vi "Pass Ref and Receive Data.vi"(7 "Enum State":T1=enum."Pass Data", 8 "error in (no error)":errorcluster, 10 "Data":T2={"Raw Data"=[], "Volt Channel"={"Index"=[], "Chl Name"=[], "Scale"=[], "Offset"=[], "Sample Rate"=100, "Device Name"="", "Channel"=""}}, 11 "Graph Manager in":refnum<class "Display Abstract.lvclass">) -> (0 "error out":errorcluster, 2 "Data Out":waveform(dbl)[](array[waveform]), 3 "Graph Manager out":refnum<class "Display Abstract.lvclass">)   [LabVIEW 2021, in "Display Abstract.lvclass"]
doc: "Do nothing."
uses:
  Display Abstract.lvclass
  Graph Data -- cluster.ctl
  Control/Volt Chl.ctl
  Pass Ref and Receive Data -- Enum.ctl
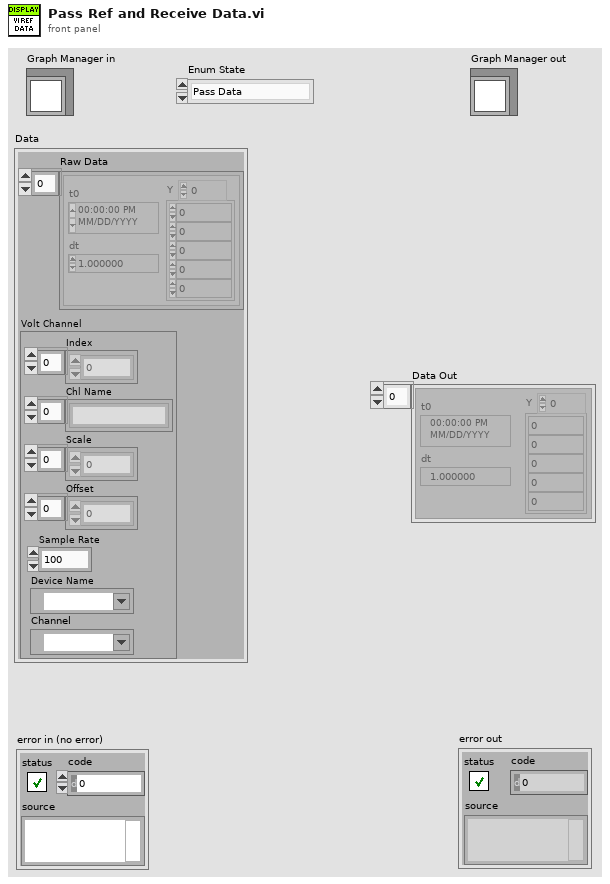
[diagram p1: front panel]
types:
  T1 = typedef "Pass Ref and Receive Data -- Enum.ctl" = enum16{"Initialize", "Pass Data"}
  T2 = typedef "Graph Data -- cluster.ctl" = cluster{"Raw Data":waveform(dbl)[], "Volt Channel":T3}
  T3 = typedef "Volt Chl.ctl" = cluster{"Index":i32[], "Chl Name":string[], "Scale":dbl[], "Offset":dbl[], "Sample Rate":i32, "Device Name":tag, "Channel":tag}
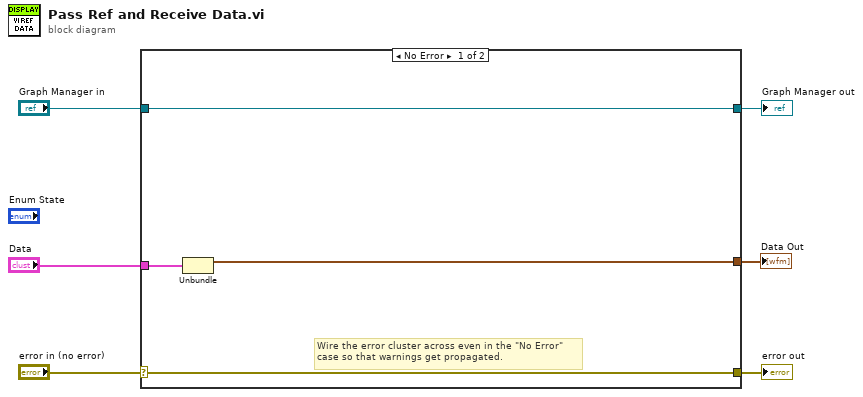
[diagram p0: block diagram]
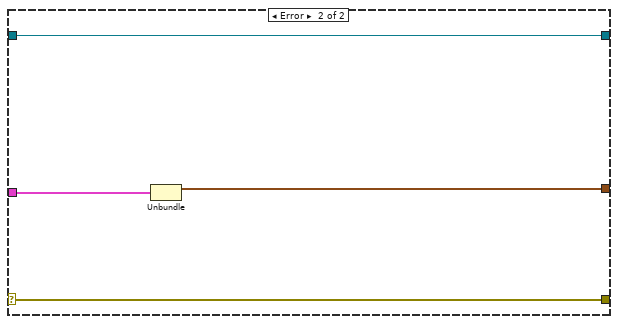
[diagram p2: hidden frame]
diagram:
  n1 = case shown="No Error" "error in (no error)" {
    selector: "error in (no error)" -> [w9 w14]
    tunnel: [w9 w14] -> w5
    tunnel: [w10 w13] -> w3
    tunnel: "Graph Manager in" -> [w10 w13]
    tunnel: "Data" -> [w8 w12]
    tunnel: [w7 w11] -> w1
    frame No Error {
      # "Wire the error cluster across even in the \"No Error\"\ncase so that warnings get propagated."
      n2 = Unbundle(w8) -> ("Raw Data"=w7:waveform(dbl)[])  [unwired: 1 out]
    }
    frame Error {
      n3 = Unbundle(w12) -> ("Raw Data"=w11:waveform(dbl)[])  [unwired: 1 out]
    }
  }
  "error out" <- w5
  "Graph Manager out" <- w3
  "Data Out" <- w1
